vi "verify expouse time.vi"(8 "error in (no error)":errorcluster, 11 "Simulated_CCD_Camera in":refnum<class "Sim_Ixon_Ultra.lvclass">) -> (0 "error out":errorcluster, 3 "Simulated_CCD_Camera out":refnum<class "Sim_Ixon_Ultra.lvclass">)   [LabVIEW 2018, in "Sim_Ixon_Ultra.lvclass"]
uses:
  Sim_Ixon_Ultra.lvclass
  Sim_Ixon_Ultra.lvclass/Sim_Ixon_Ultra.ctl
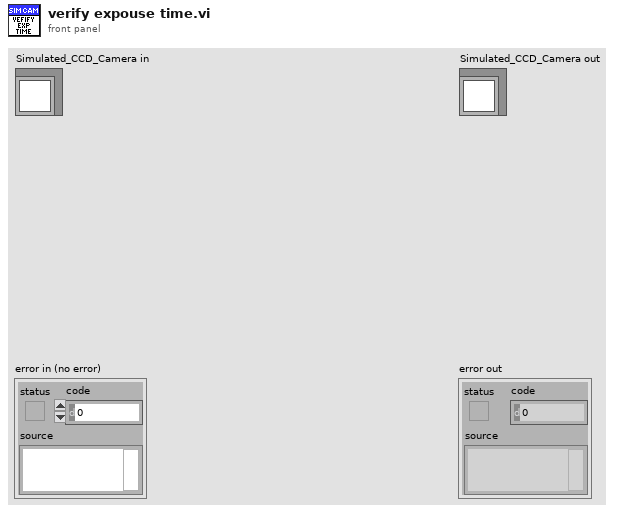
[diagram p1: front panel]
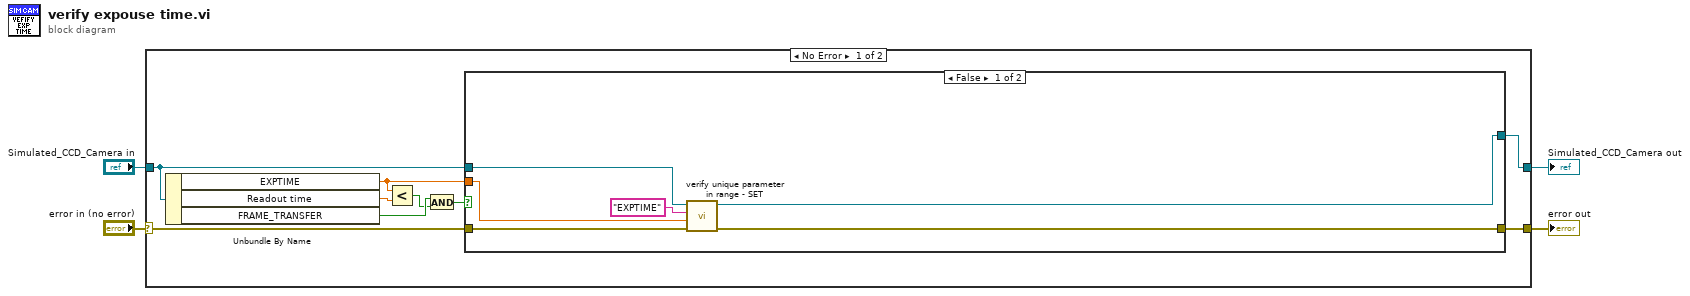
[diagram p0: block diagram]
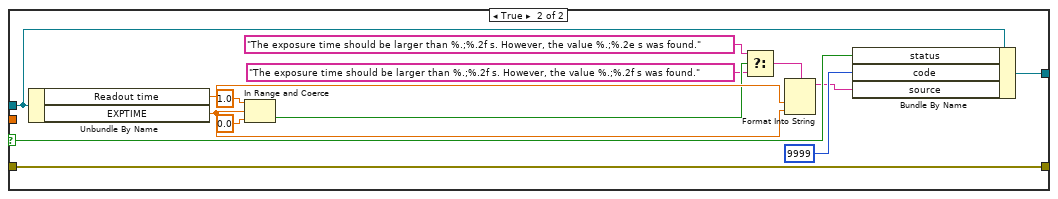
[diagram p2: hidden frame]
diagram:
  n1 = case shown="No Error" "error in (no error)" {
    selector: "error in (no error)" -> [w8 w35]
    tunnel: [w6 w35] -> w3
    tunnel: [w9 w34] -> w2
    tunnel: "Simulated_CCD_Camera in" -> [w5 w34]
    frame No Error {
      n2 = Unbundle By Name(w5) -> ("EXPTIME"=w7:dbl, "Readout time"=w12:dbl, "FRAME_TRANSFER"=w13:bool)
      n3 = Less?(x=w7, y=w12) -> (x < y?=w11:bool)
      n4 = And(x=w13, y=w11) -> (x .and. y?=w10:bool)
      n5 = case shown="False" w10 {
        selector: w10 -> [_ w32]
        tunnel: [w15 w33] -> w9
        tunnel: w8 -> [w19 w20]
        tunnel: w7 -> [w18 _]
        tunnel: w5 -> [w17 w21]
        tunnel: [w16 w20] -> w6
        frame False {
          n6 = call "verify unique parameter in range - SET.vi"("error in (no error)"=w19, "value"=w18, "parameter name"="EXPTIME", "Simulated_CCD_Camera in"=w17) -> ("error out"=w16:errorcluster, "Simulated_CCD_Camera out"=w15:refnum<class "Sim_Ixon_Ultra.lvclass">)  [unwired: 6 in]
        }
        frame True {
          n7 = Unbundle By Name(w21) -> ("Readout time"=w29:dbl, "EXPTIME"=w27:dbl)
          n8 = In Range and Coerce(upper limit=1.0, x=w27, lower limit=0.0 ("upper limit")) -> (In Range?=w26:bool)  [unwired: 1 out]
          n9 = Select(t="The exposure time should be larger than %.;%.2f s. However, the value %.;%.2e s was found." ("format string"), s=w26, f="The exposure time should be larger than %.;%.2f s. However, the value %.;%.2f s was found." ("format string")) -> (s? t:f=w23:string)
          n10 = Format Into String(format string=w23, w29, w27) -> (resulting string=w30:string)  [unwired: 2 in, 1 out]
          n11 = Bundle By Name(cluster=w21, "status"=w32, "code"=9999 ("SET errors.exposure time.code"), "source"=w30) -> (w33:refnum<class "Sim_Ixon_Ultra.lvclass">)
        }
      }
    }
    frame Error {
    }
  }
  "error out" <- w3
  "Simulated_CCD_Camera out" <- w2
